vi "New Parent.vi"(8 "error in (no error)":errorcluster, 10 "ToPanel:New":refnum<user-event>, 11 "TipPanel in":refnum<class "TipPanel.lvclass">) -> (0 "error out":errorcluster, 3 "TipPanel out":refnum<class "TipPanel.lvclass">)   [LabVIEW 2021, in "TipStripOOPanel.lvlib" / "TipPanel.lvclass"]
uses:
  TipPanel.lvclass
  ToPanelUEWrapper.ctl
  ToPanelUE.ctl
  <vilib>/Futures/Futures/Promise/Promise.lvclass
  TipPanel.lvclass/TipPanel.ctl
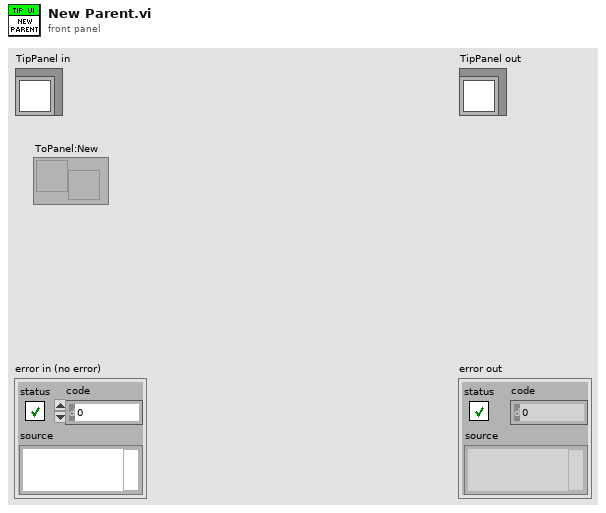
[diagram p1: front panel]
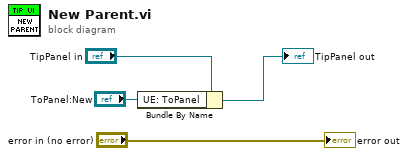
[diagram p0: block diagram]
diagram:
  n1 = Bundle By Name(cluster="TipPanel in", "UE: ToPanel"="ToPanel:New") -> (→"TipPanel out":refnum<class "TipPanel.lvclass">)
  "error out" <- "error in (no error)"
